vi "Flush.vi"(8 "error in (no error)":errorcluster, 11 "Priority Queue in":refnum<class "Message Priority Queue.lvclass">) -> (0 "error out":errorcluster, 2 "remaining elements":refnum<class "Message.lvclass">[](array[class]), 3 "Priority Queue out":refnum<class "Message Priority Queue.lvclass">)   [LabVIEW 2017, in "Actor Framework.lvlib" / "Message Priority Queue.lvclass"]
uses:
  <vilib>/ActorFramework/Message Priority Queue/Message Priority Queue.lvclass
  <vilib>/ActorFramework/Message/Message.lvclass
  <vilib>/ActorFramework/Message Priority Queue/Message Priority Queue.lvclass/Message Priority Queue.ctl
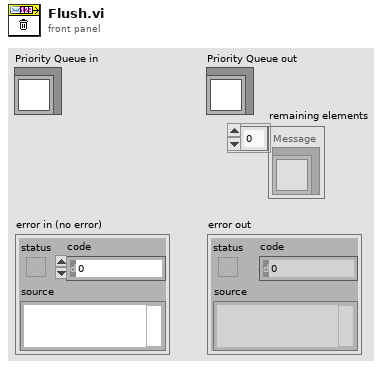
[diagram p1: front panel]
types:
  T1 = typedef "Actor Framework.lvlib/Message Priority Queue.lvclass/DVR Contents.ctl" = cluster{"# Waiting":u32, "Buffers":refnum<queue>[], "Wait Msg":refnum<queue>, "Wait Prior":refnum<queue>}
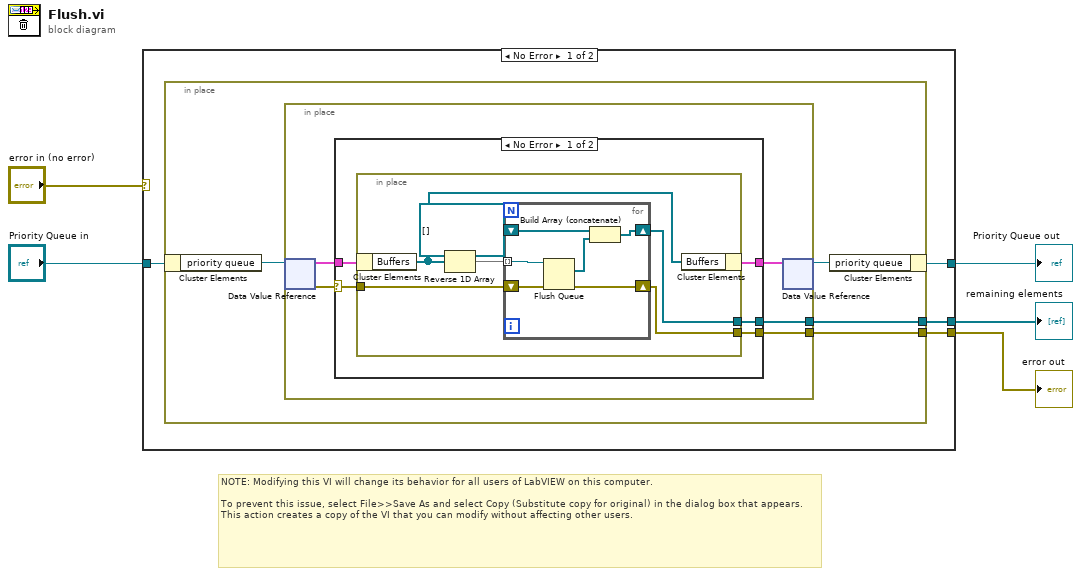
[diagram p0: block diagram]
diagram:
  # "NOTE: Modifying this VI will change its behavior for all users of LabVIEW on this computer.\n\nTo prevent this issue, select File>>Save As and select Copy (Substitute copy for original) in the dialog box that appears. This action creates a copy of the VI that you can modify without affecting other users."
  n1 = case shown="No Error" "error in (no error)" {
    selector: "error in (no error)" -> [_ w39]
    tunnel: "Priority Queue in" -> [w9 w38]
    tunnel: [w8 w39] -> w3
    tunnel: [w7 _] -> w2
    tunnel: [w6 w38] -> w1
    frame No Error {
      n2 = in-place {
        in-place-border: [w11] -> w8
        in-place-border: [w10] -> w7
        n3 = in-place-cluster #1(w9) -> ("priority queue"=w13:refnum<data-value>)
        n4 = in-place {
          in-place-border: [w15] -> w11
          in-place-border: [w14] -> w10
          n5 = in-place-dvr #2(w13) -> (w17:T1, w18:errorcluster)
          n6 = case shown="No Error" w18 {
            selector: w18 -> [w21 w36]
            tunnel: w17 -> [w23 w37]
            tunnel: [w22 w37] -> w16
            tunnel: [w20 w36] -> w15
            tunnel: [w19 _] -> w14
            frame No Error {
              n7 = in-place {
                in-place-border: w21 -> [w28]
                in-place-border: [w27] -> w20
                in-place-border: [w25] -> w19
                n8 = in-place-cluster #3(w23) -> ("Buffers"=w29:refnum<queue>[])
                n9 = Reverse 1D Array(array=w29) -> (reversed array=w24:refnum<queue>[])
                n10 = for {
                  tunnel: w24 -> [w35] mode=indexing
                  shift-right: [w33] -> w27
                  shift-left: w28 -> [w34]
                  shift-right: [w32] -> w25
                  shift-left: refnum<class "Message.lvclass">[] [] -> [w30]
                  n11 = Flush Queue(queue=w35, error in (no error)=w34) -> (remaining elements=w31:refnum<class "Message.lvclass">[], error out=w33:errorcluster)  [unwired: 1 out]
                  n12 = Build Array (concatenate)(w30, w31) -> (w32:refnum<class "Message.lvclass">[])
                }
                n13 = in-place-cluster #3("Buffers"=w29) -> (w22:T1)
              }
            }
            frame Error {
            }
          }
          n14 = in-place-dvr #2(w16) -> (w12:refnum<data-value>)  [unwired: 1 out]
        }
        n15 = in-place-cluster #1("priority queue"=w12) -> (w6:refnum<class "Message Priority Queue.lvclass">)
      }
    }
    frame Error {
    }
  }
  "Priority Queue out" <- w1
  "error out" <- w3
  "remaining elements" <- w2
